vi "onetest.000000.vi"(7 "N":dbl=100.0) -> ()   [LabVIEW 2016]
panel:
  out "XY Graph":cluster{i32[], dbl[]}(graph)={[0, 1, 2, 3, 4, 5, 6, 7, 8, 9, 10, 11, 12, 13, 14, 15, 16, 17, 18, 19, 20, 21, 22, 23, 24, 25, 26, 27, 28, 29, 30, 31, 32, 33, 34, 35, 36, 37, 38, 39, 40, 41, 42, 43, 44, 45, 46, 47, 48, 49, 50, 51, 52, 53, 54, 55, 56, 57, 58, 59, 60, 61, 62, 63, 64, 65, 66, 67, 68, 69, 70, 71, 72, 73, 74, 75, 76, 77, 78, 79, 80, 81, 82, 83, 84, 85, 86, 87, 88, 89, 90, 91, 92, 93, 94, 95, 96, 97, 98, 99], [0.17854993035965627, 0.8905754231799967, 0.1056823112245624, 0.9515489573915334, 0.21982681151186512, 0.7769292663644309, 0.7660701636255756, 0.055521704959712315, 0.6847338907095433, 0.25441788083139905, 0.035678803731361786, 0.10078736707079772, 0.4687706139766732, 0.6557197431097237, 0.7552776247791764, 0.2308243646995467, 0.8934365545392264, 0.2930331781182536, 0.3410554059563593, 0.015130679491307308, 0.3116356681809378, 0.2476294751573993, 0.7325203024390639, 0.03642681023205441, 0.8219490921157468, 0.0402444955911927, 0.13540034213675334, 0.4712756834572538, 0.263348480002493, 0.9789634547540872, 0.021203116465263072, 0.17897247287007367, 0.26540464279870823, 0.7597676205446593, 0.4579630349324282, 0.4300067550306421, 0.6535431066309916, 0.7082324417679489, 0.1902661541071986, 0.7151595119870566, 0.8873964728613383, 0.3928622061080169, 0.5112351534789736, 0.4653551328660577, 0.9020780060674416, 0.09985284226272473, 0.4161954354139843, 0.33068684676339344, 0.35179431758945157, 0.7838004830189078, 0.4498110438066303, 0.8668140494934506, 0.11833644416285205, 0.25602109460109457, 0.5492959088533775, 0.06061267064058473, 0.47243285944417357, 0.809466202899513, 0.2785756755972688, 0.10960607553981694, 0.4056476890871039, 0.7541193658184278, 0.398594672110699, 0.29140155172047133, 0.9610359091841736, 0.9888417673134439, 0.6984656032791223, 0.12269944667462296, 0.5354032046862767, 0.1760025551114921, 0.7907402641309875, 0.7931755796299251, 0.39728191673057367, 0.8076924889092538, 0.6071201818720986, 0.5270707402670116, 0.34294139786331446, 0.4236271684285198, 0.5995987062791259, 0.8786399221006004, 0.5317971553580707, 0.2760380702451636, 0.05356760064692434, 0.9172576532672498, 0.8888608041469119, 0.45567126574596806, 0.06854033244573321, 0.34158350238314966, 0.29287438747300887, 0.26040668235211095, 0.23686598302077488, 0.7696005413502649, 0.27534301180140064, 0.7420199215956857, 0.5073115142749018, 0.8519720806479737, 0.969797441595247, 0.6750640171501805, 0.21879227414682179, 0.27459808746236924]}
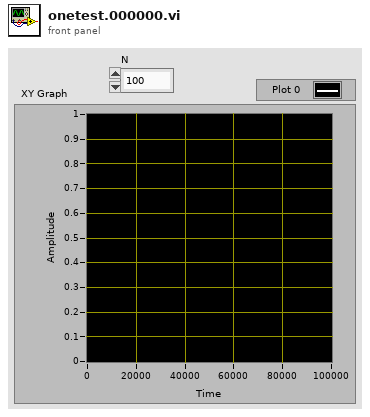
[diagram p1: front panel]
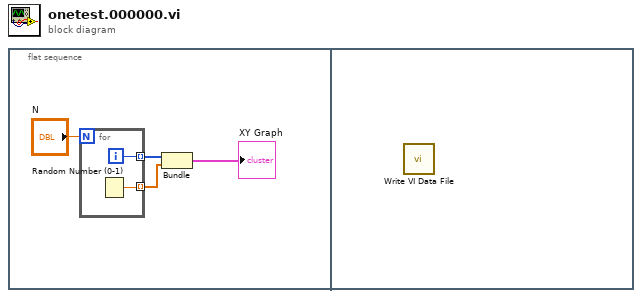
[diagram p0: block diagram]
diagram:
  n1 = flat-sequence {
    frame #0 {
      n2 = for {
        N: "N" -> [_]
        tunnel: [w6] -> w3 mode=indexing
        tunnel: [w5] -> w4 mode=indexing
        i -> [w5]
        n3 = Random Number (0-1)() -> (number: 0 to 1=w6:dbl)
      }
      n4 = Bundle(w4, w3) -> (→"XY Graph":cluster{i32[], dbl[]})  [unwired: 1 in]
    }
    frame #1 {
      n5 = call "Write VI Data File.vi"() -> ()  [unwired: 10 in, 2 out]
    }
  }
